vi "Test Method 2.vi"(11 "Test Case In":refnum<class "My Test Case.lvclass">) -> (0 "error out":errorcluster, 3 "Test Case Out":refnum<class "My Test Case.lvclass">)   [LabVIEW 2020, in "My Test Case.lvclass"]
uses:
  My Test Case.lvclass
  My Test Case.lvclass/My Test Case.ctl
  4993e8ee-a06a-463a-9684-69129f64d5ce.vi
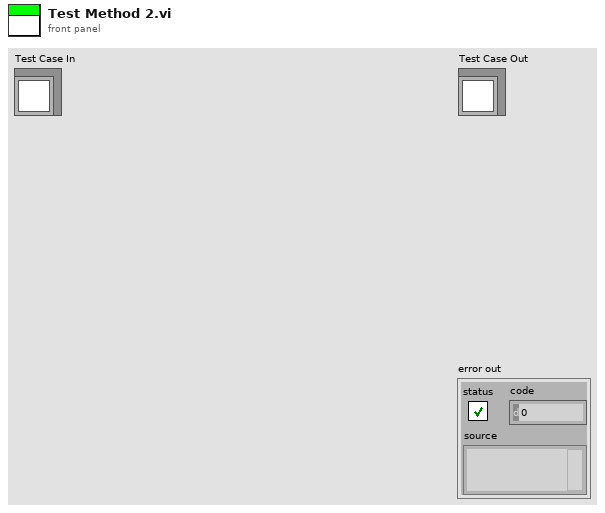
[diagram p1: front panel]
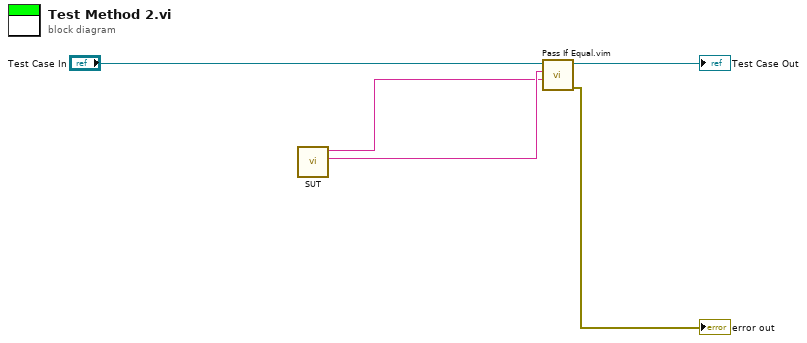
[diagram p0: block diagram]
diagram:
  n1 = call "SUT.vi"() -> ("String 2"=w2:string, "String"=w1:string)  [unwired: 10 in]
  n2 = call "Pass If Equal.vim"("Actual"=w1, "Expected"=w2, "LUnit Test Case In"="Test Case In") -> ("error out"=→"error out":errorcluster, "LUnit Test Case Out"=→"Test Case Out":refnum<class "My Test Case.lvclass">)  [unwired: 7 in]
